vi "WriteLeftData.vi"(8 "error in (no error)":errorcluster, 10 "Left":T1, 11 "MAUI in":refnum<class "MAUI.lvclass">) -> (0 "error out":errorcluster, 3 "MAUI out":refnum<class "MAUI.lvclass">)   [LabVIEW 2016, in "MAUI.lvclass"]
uses:
  MAUI.lvclass
  Typedefs/PrivateEvents--MAUI.SetLeftData.ctl
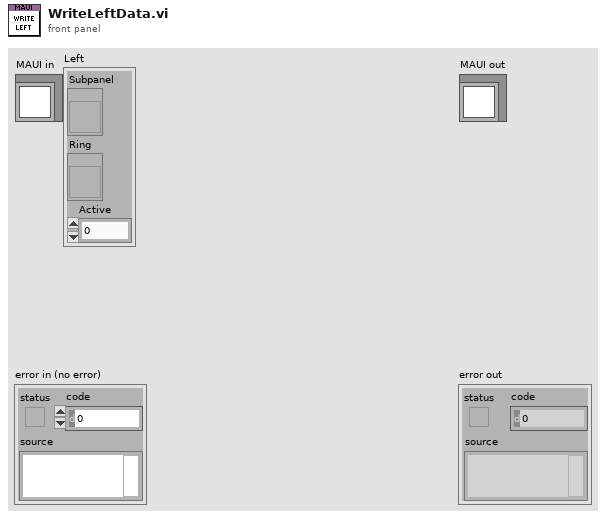
[diagram p1: front panel]
types:
  T1 = cluster{"Subpanel":refnum<vi>, "Ring":refnum<vi>, "Active":i32}
  T2 = typedef "MAUI.lvclass/PrivateEvents--MAUI.SetLeftData.ctl" = cluster{"Left":cluster{"Subpanel":refnum<vi>, "Ring":refnum<vi>, "Active":i32}}
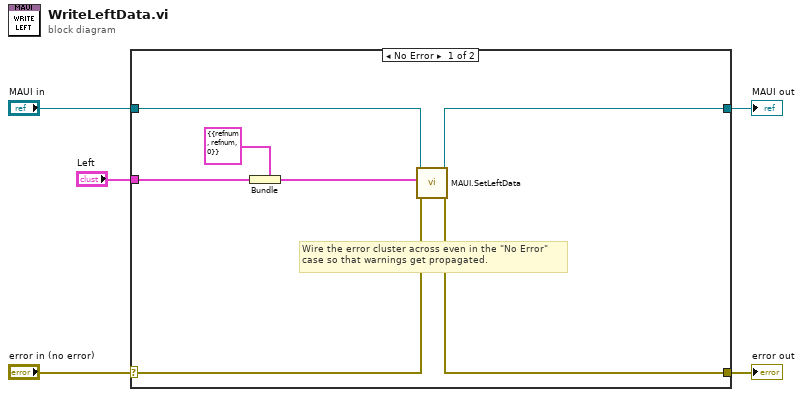
[diagram p0: block diagram]
diagram:
  n1 = case shown="No Error" "error in (no error)" {
    selector: "error in (no error)" -> [w12 w14]
    tunnel: [w11 w14] -> w4
    tunnel: [w9 w13] -> w2
    tunnel: "MAUI in" -> [w10 w13]
    tunnel: "Left" -> [w6 _]
    frame No Error {
      # "Wire the error cluster across even in the \"No Error\"\ncase so that warnings get propagated."
      n2 = Bundle(cluster=T2 {"Left"={"Subpanel"=refnum, "Ring"=refnum, "Active"=0}} ("SetLeftData"), "Left"=w6) -> (w8:T2)
      n3 = call "MAUI.SetLeftData.vi"("error in (no error)"=w12, "SetLeftData"=w8, "MAUI"=w10) -> ("error out"=w11:errorcluster, "MAUI out"=w9:refnum<class "MAUI.lvclass">)  [unwired: 7 in]
    }
    frame Error {
    }
  }
  "error out" <- w4
  "MAUI out" <- w2
